vi "API POST Multipart File Upload.vi"(0 "DocumentRevisionId":string, 1 "XY Parallel":string, 2 "Python Version":enum32{"2.7", "3.6"}(radio), 3 "XY Series":string, 5 "API Token":string="apitoken 475eef11-95b9-4f32-9221-3162004815ef:f20a91a0-c04e-4d32-b0b4-337e6e91bde7", 7 "Select environment":enum32{"dev.", "demo.", ""}(radio), 9 "Paths":string[](array[string]), 11 "POST/PATCH error in (no error)":errorcluster, 12 "FormInput Names":string, 13 "Python file path":path, 14 "FormInput Values":string) -> (4 "Updated formInput":string, 6 "Assigned attachments":string, 10 "POST/PATCH Request error out":errorcluster, 15 "POST/PATCH error out":errorcluster)   [LabVIEW 2019]
uses:
  <vilib>/LVH/i3 JSON/JSON Parsing/Get Object Parameter Files/Get Object Parameter - Numeric.vi
  <vilib>/LVH/i3 JSON/JSON Parsing/Get Object Parameter Files/Get Object Parameter - String.vi
  <vilib>/LVH/i3 JSON/JSON Parsing/Get Object Parameter Files/Get Object Parameter - Object.vi
  <vilib>/LVH/i3 JSON/i3-json.lvlib
panel:
  in  "error in (no error)":errorcluster
  out "Status":string
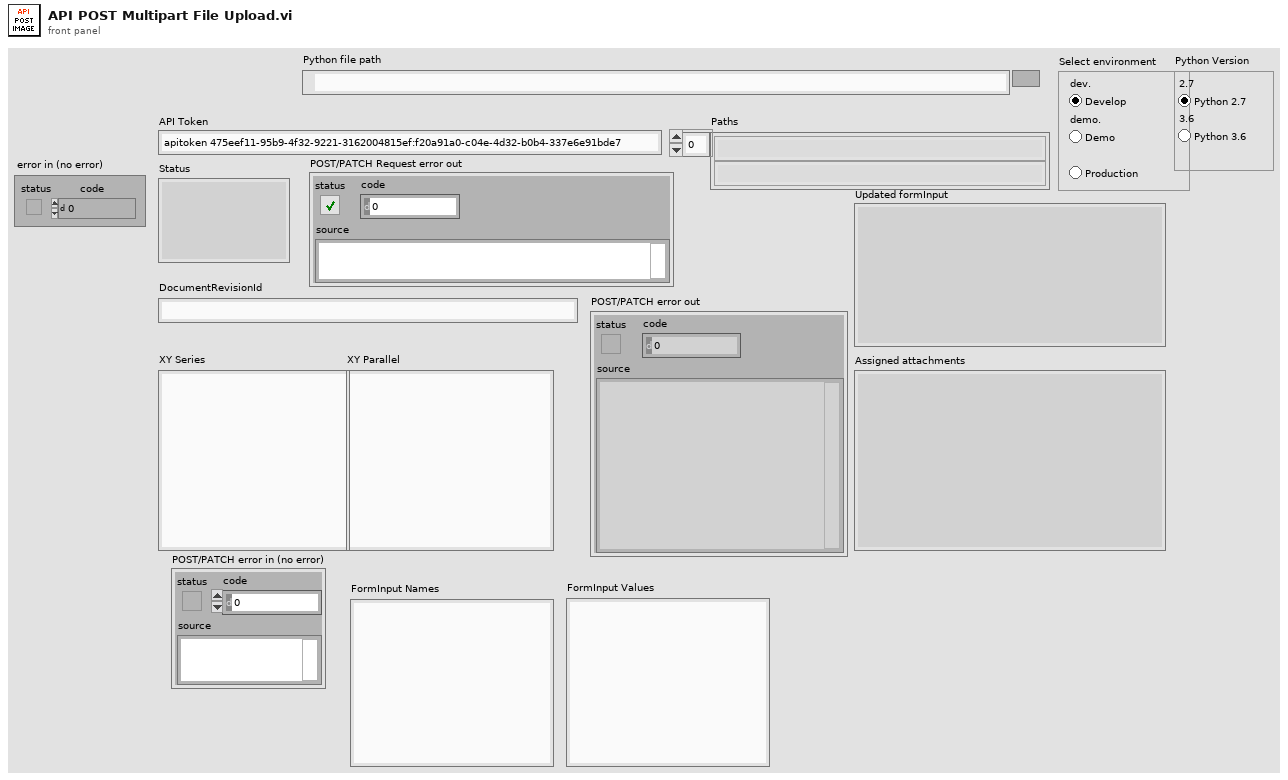
[diagram p1: front panel]
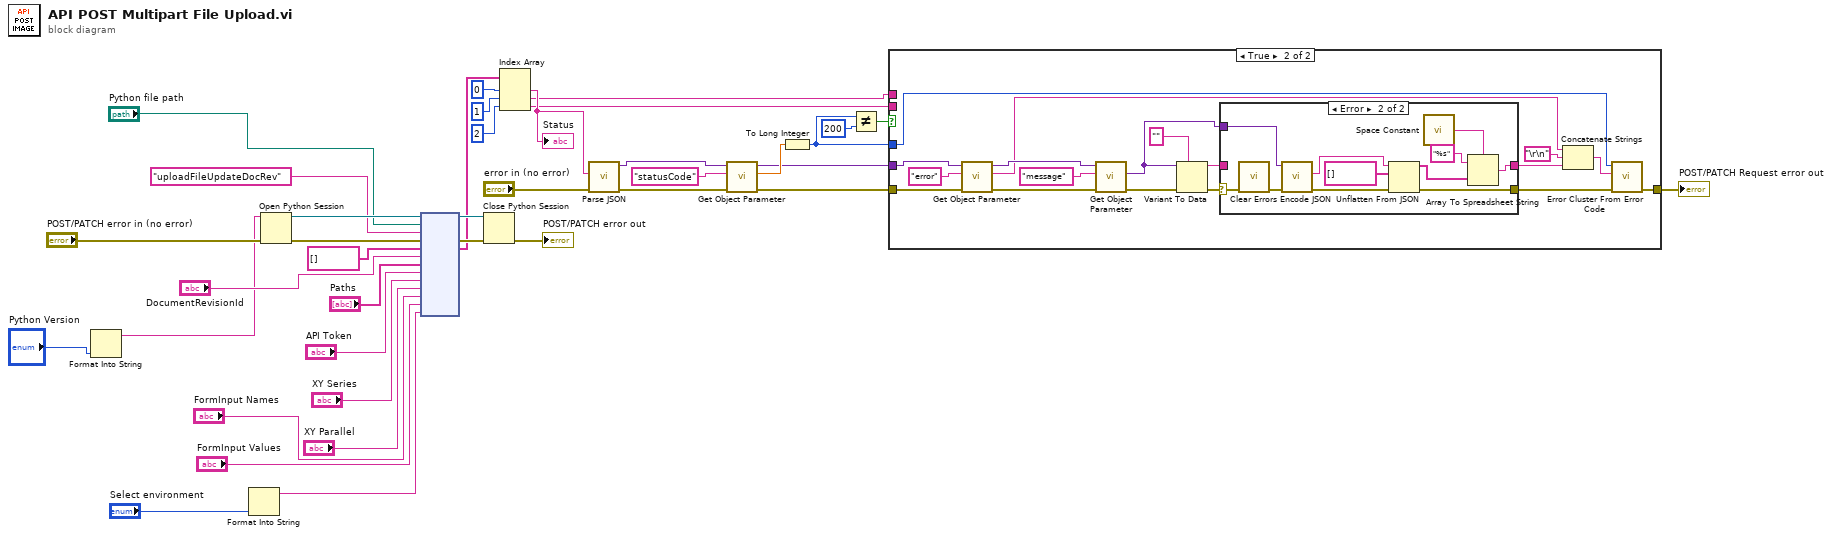
[diagram p0: block diagram]
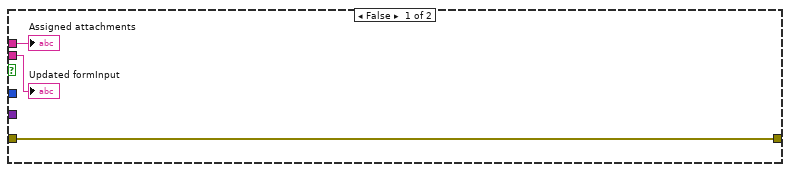
[diagram p2: hidden frame]
diagram:
  n1 = Format Into String("Python Version") -> (resulting string=w2:string)  [unwired: 3 in, 1 out]
  n2 = Format Into String("Select environment") -> (resulting string=w4:string)  [unwired: 3 in, 1 out]
  n3 = Open Python Session(python version=w2, 3:"POST/PATCH error in (no error)") -> (session out=w38:refnum<k35>, error out=w37:errorcluster)  [unwired: 1 in]
  n4 = node(w38, "Python file path", "uploadFileUpdateDocRev" ("function name"), w37, string[] [], "DocumentRevisionId", "Paths", "API Token", "XY Series", "XY Parallel", "FormInput Names", "FormInput Values", w4) -> (w34:refnum<k35>, w36:errorcluster, w23:string[])  [unwired: 8 in, 2 out]
  n5 = Close Python Session(session in=w34, error in=w36) -> (11:→"POST/PATCH error out":errorcluster)
  n6 = Index Array(array=w23, index #1=0 ("index"), index #2=1 ("index"), index #3=2 ("index")) -> (element #1=w8:string, element #2=w6:string, element #3=w7:string)
  "Status" <- w8
  n7 = call <vilib>:"Parse JSON.vi"("error in (no error)"="error in (no error)", "JSON String"=w8) -> ("error out"=w13:errorcluster, "JSON Tree"=w15:variant)  [unwired: 6 in, 2 out]
  n8 = call-poly <vilib>:"Get Object Parameter.vi"("error in (no error)"=w13, "Parameter Name"="statusCode", "JSON Tree In (JSON Object)"=w15) -> ("error out"=w12:errorcluster, "Double Value"=w18:dbl, "JSON Tree Out Passthrough"=w11:variant)  [unwired: 5 in, 1 out]
  n9 = To Long Integer(number=w18) -> (32bit integer=w10:i32)
  n10 = Not Equal?(x=w10, y=200) -> (x != y?=w16:bool)
  n11 = case shown="True" w16 {
    tunnel: w11 -> [_ w45]
    tunnel: w12 -> [w41 w44]
    tunnel: w10 -> [_ w43]
    tunnel: [w41 w42] -> w9
    tunnel: w7 -> [w40 _]
    tunnel: w6 -> [w39 _]
    frame False {
      "Updated formInput" <- w40
      "Assigned attachments" <- w39
    }
    frame True {
      n12 = call-poly <vilib>:"Get Object Parameter.vi"("error in (no error)"=w44, "Parameter Name"="error", "JSON Tree In (JSON Object)"=w45) -> ("error out"=w56:errorcluster, "String Value"=w55:string, "JSON Tree Out Passthrough"=w57:variant)  [unwired: 5 in, 1 out]
      n13 = call-poly <vilib>:"Get Object Parameter.vi"("error in (no error)"=w56, "Parameter Name"="message", "JSON Tree In (JSON Object)"=w57) -> ("error out"=w51:errorcluster, "JSON Object"=w48:variant)  [unwired: 5 in, 2 out]
      n14 = Variant To Data(error in=w51, type="", Variant=w48) -> (data=w49:string, error out=w50:errorcluster)
      n15 = case shown="Error" w50 {
        selector: w50 -> [w60 w65]
        tunnel: w49 -> [w61 _]
        tunnel: [w61 w62] -> w47
        tunnel: w48 -> [_ w66]
        tunnel: [w60 w63] -> w46
        frame No Error {
        }
        frame Error {
          n16 = call <vilib>:"Clear Errors.vi"("error in (no error)"=w65) -> ("error out"=w64:errorcluster)  [unwired: 5 in, 1 out]
          n17 = call <vilib>:"Encode JSON.vi"("error in (no error)"=w64, "JSON Tree"=w66) -> ("error out"=w70:errorcluster, "String"=w69:string)  [unwired: 4 in]
          n18 = Unflatten From JSON(JSON string=w69, type and defaults=string[] [], error in (no error)=w70) -> (value=w71:string[], error out=w63:errorcluster)  [unwired: 4 in]
          n19 = call <vilib>:"Space Constant.vi"() -> ("String"=w72:string)
          n20 = Array To Spreadsheet String(delimiter (Tab)=w72, array=w71, 3:"%s" ("format string")) -> (spreadsheet string=w62:string)
        }
      }
      n21 = Concatenate Strings(w55, "\r\n", w47) -> (w54:string)
      n22 = call <vilib>:"Error Cluster From Error Code.vi"("error in (no error)"=w46, "error message (\"\")"=w54, "error code (0)"=w43) -> ("error out"=w42:errorcluster)  [unwired: 6 in]
    }
  }
  "POST/PATCH Request error out" <- w9
